vi "ExTestKineticsNew.vi"() -> ()   [LabVIEW 2010]
panel:
  in  "Enum":T1(ring)
  in  "Window Size":u32=10 min=1 step=1
  out "Boolean":bool
  out "x Size":u32
  out "x post":u32
  out "x pre":u32
  out "y Size":u32
  out "y post":u32
  out "y pre":u32
  in  "Software Accumulation":u32=1 min=1 step=1
  in  "Intensifier":bool
  in  "Temperature":dbl=-10.0 format="%.2f"
  in  "Exposure":dbl min=0.0 step=1e-06 format="%.5f"
  in  "stop":bool
  in  "Store":bool
  out "error out":errorcluster
  in  "error in (no error)":errorcluster
  # "ExCircularBufBin2x:\nThis example only works with cameras with circualar \nbuffer capability. This routine will continously display an \nimage binned by 2 in both the x and the y direction. It \nwill store in append mode the frames while the store \ntoggle switch is on."
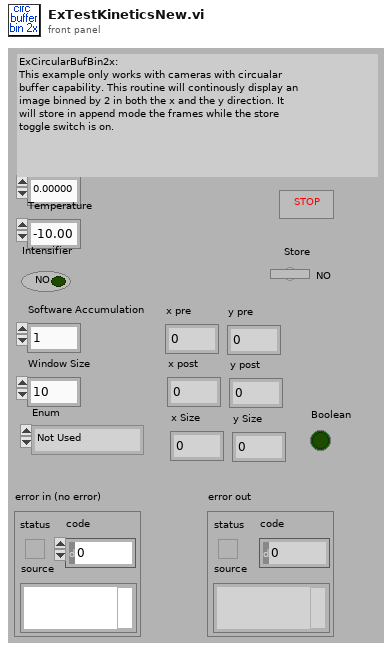
[diagram p1: front panel]
types:
  T1 = enum32{"Not Used", "No Trigger", "Single Trigger", "Multiple Trigger"}
  T2 = cluster{"Pre Y":u32, "Post Y":u32, "Parallel (Y) Size":u32, "Pre X":u32, "Post X":u32, "Serial (X) Size":u32}
  T3 = cluster{"Camera Handle":u32, "Pulser Handle":u32, "File Handle":u32, "Display Handle":u32, "Image Handle":u32}
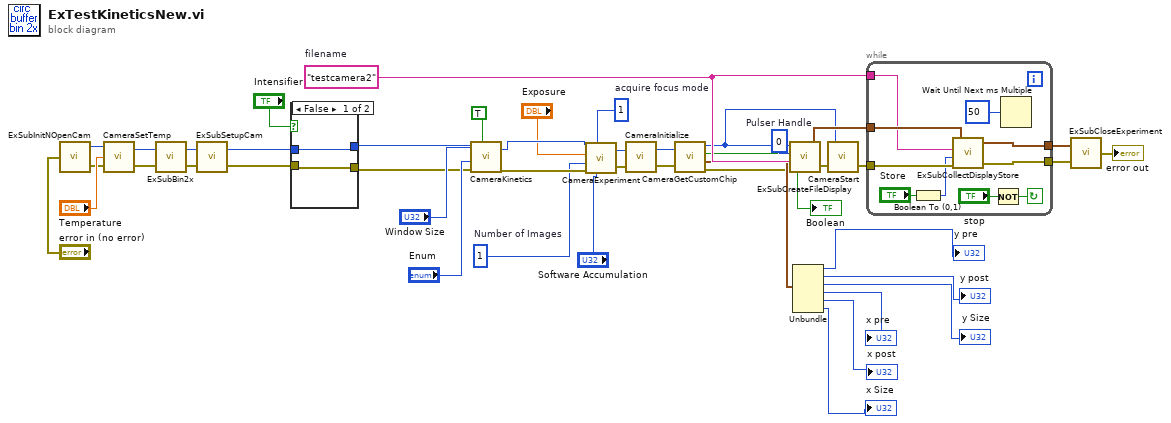
[diagram p0: block diagram]
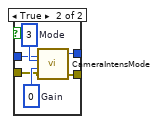
[diagram p2: hidden frame]
diagram:
  w35 = u32 0  # Pulser Handle
  w5 = u32 1  # acquire focus mode
  w4 = u32 1  # Number of Images
  w44 = "testcamera2"  # filename
  n1 = call "ExSubInitNOpenCam.vi"("error in (no error)"="error in (no error)") -> ("Camera Handle"=w33:u32, "error out"=w31:errorcluster)
  n2 = call <userlib>:"CameraSetTemp.vi"("error in (no error)"=w31, "Temperature"="Temperature", "Camera Handle"=w33) -> ("error out"=w19:errorcluster, "Camera Handle"=w20:u32)
  n3 = call "ExSubBin2x.vi"("error in (no error)"=w19, "Camera Handle"=w20) -> ("error out"=w30:errorcluster, "Camera Handle"=w36:u32)
  n4 = call "ExSubSetupCam.vi"("error in (no error)"=w30, "Camera Handle"=w36) -> ("error out"=w17:errorcluster, "Camera Handle"=w18:u32)
  n5 = case shown="False" "Intensifier" {
    tunnel: [w46 w52] -> w2
    tunnel: [w45 w51] -> w1
    tunnel: w18 -> [w46 w48]
    tunnel: w17 -> [w45 w47]
    frame False {
    }
    frame True {
      w49 = u32 0  # Gain
      w50 = u32 3  # Mode
      n6 = call <userlib>:"CameraIntensMode.vi"("error in"=w47, "Intensifier Gain"=w49, "Mode"=w50, "Camera Handle"=w48) -> ("error out"=w51:errorcluster, "Camera Handle"=w52:u32)
    }
  }
  n7 = call <userlib>:"CameraKinetics.vi"("Camera Handle"=w2, "Window Size"="Window Size", "TriggerMode"="Enum", "error in (no error)"=w1, "Enable/Disable Kinetics"=TRUE) -> ("Camera Handle"=w8:u32, "error out"=w7:errorcluster)
  n8 = call <userlib>:"CameraExperiment.vi"("Number of Accumulations"="Software Accumulation", "Acquire / Focus Flag"=w5, "error in"=w7, "Number of Images"=w4, "Exposure (sec)"="Exposure", "Camera Handle"=w8) -> ("error out"=w10:errorcluster, "Camera Handle"=w9:u32)
  n9 = call <userlib>:"CameraInitialize.vi"("error in"=w10, "Camera Handle"=w9) -> ("error out"=w13:errorcluster, "Camera Handle"=w14:u32)
  n10 = call <userlib>:"CameraGetCustomChip.vi"("Camera Handle"=w14, "error in (no error)"=w13) -> ("Camera Handle"=w12:u32, "Custum chip Enable/Disable status"=→"Boolean":bool, "CameraGetCustomChip"=w29:T2, "error out"=w22:errorcluster)
  n11 = call "ExSubCreateFileDisplay.vi"("error in (no error)"=w22, "File and Display Name"=w44, "Pulser Handle"=w35, "Camera Handle"=w12) -> ("error out"=w37:errorcluster, "Handles Out"=w42:T3)
  n12 = Unbundle(w29) -> ("Pre Y"=→"y pre":u32, "Post Y"=→"y post":u32, "Parallel (Y) Size"=→"y Size":u32, "Pre X"=→"x pre":u32, "Post X"=→"x post":u32, "Serial (X) Size"=→"x Size":u32)
  n13 = call <userlib>:"CameraStart.vi"("error in"=w37, "Camera Handle"=w12) -> ("error out"=w38:errorcluster)  [unwired: 1 out]
  n14 = while {
    tunnel: w42 -> [w61]
    tunnel: w38 -> [w60]
    tunnel: w44 -> [w53]
    tunnel: [w58] -> w40
    tunnel: [w59] -> w41
    stop <- w56 continue-if-true
    n15 = Boolean To (0,1)(Boolean="Store") -> (0, 1=w54:i16)
    n16 = call "ExSubCollectDisplayStore.vi"("error in (no error)"=w60, "Store flag"=w54, "Display Title"=w53, "Handle Cluster"=w61) -> ("error out"=w58:errorcluster, "Handle Cluster Out"=w59:T3)  [unwired: 1 out]
    n17 = Not(x="stop") -> (.not. x?=w56:bool)
    n18 = Wait Until Next ms Multiple(millisecond multiple=u32 50) -> ()  [unwired: 1 out]
  }
  n19 = call "ExSubCloseExperiment.vi"("error in (no error)"=w40, "Handles In"=w41) -> ("error out"=→"error out":errorcluster)
